vi "UE9 Config Comm.vi"() -> ()   [LabVIEW 2021]
panel:
  in  "Power Level":u8
  in  "Local ID":u8=1
  in  "DHCP Enabled":bool
  in  "Subnet":string="255.255.255.0"
  in  "Gateway":string="192.168.1.1"
  in  "PortB":u16=52361
  in  "PortA":u16=52360
  in  "IP Address":string="192.168.1.209"
  in  "FirstFound":bool=TRUE
  in  "ConnectionType":string="LJ_ctUSB"
  in  "Address":string="192.168.1.209"
  out "Error Message":string
  in  "error in":errorcluster
  out "error out":errorcluster
  # "Specify an IP address for Ethernet, or Local ID\nfor USB.  If FirstFound is selected, Local ID is\nignored for USB."
  # "Reset required for Ethernet parameters\nto take effect."
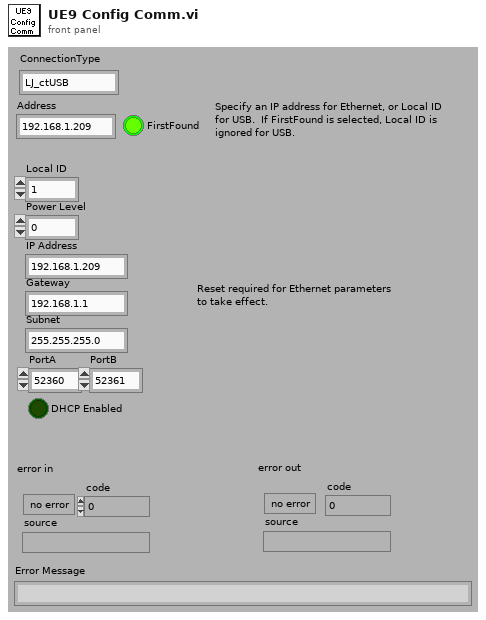
[diagram p1: front panel]
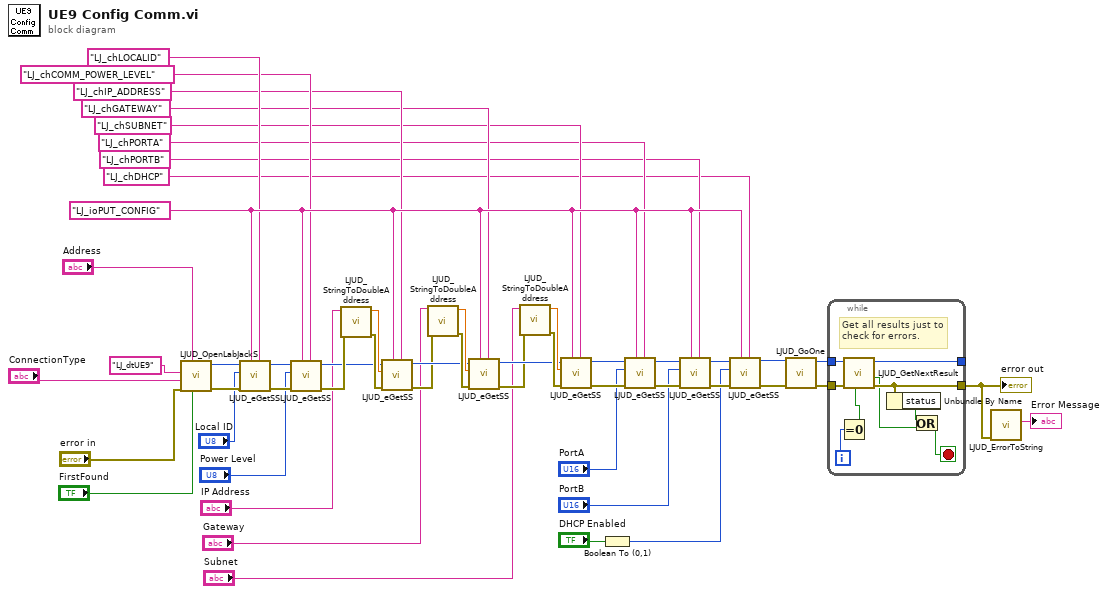
[diagram p0: block diagram]
diagram:
  w22 = "LJ_ioPUT_CONFIG" ("IOType")
  n1 = call "LJUD_OpenLabJackS.vi"("FirstFound"="FirstFound", "Address"="Address", "error in"="error in", "ConnectionType"="ConnectionType", "DeviceType"="LJ_dtUE9") -> ("error out"=w35:errorcluster, "Handle"=w38:i32)  [unwired: 4 in, 1 out]
  n2 = call "LJUD_eGetSS.vi"("Channel"="LJ_chLOCALID", "IOType"=w22, "error in"=w35, "Value Write"="Local ID", "Handle In"=w38) -> ("error out"=w34:errorcluster, "Handle Out"=w37:i32)  [unwired: 4 in, 1 out]
  n3 = call "LJUD_eGetSS.vi"("Channel"="LJ_chCOMM_POWER_LEVEL", "IOType"=w22, "error in"=w34, "Value Write"="Power Level", "Handle In"=w37) -> ("error out"=w28:errorcluster, "Handle Out"=w27:i32)  [unwired: 4 in, 1 out]
  n4 = call "LJUD_StringToDoubleAddress.vi"("error in"=w28, "String"="IP Address") -> ("error out"=w32:errorcluster, "Double Address"=w47:dbl)  [unwired: 8 in]
  n5 = call "LJUD_eGetSS.vi"("Channel"="LJ_chIP_ADDRESS", "IOType"=w22, "error in"=w32, "Value Write"=w47, "Handle In"=w27) -> ("error out"=w40:errorcluster, "Handle Out"=w42:i32)  [unwired: 4 in, 1 out]
  n6 = call "LJUD_StringToDoubleAddress.vi"("error in"=w40, "String"="Gateway") -> ("error out"=w45:errorcluster, "Double Address"=w46:dbl)  [unwired: 8 in]
  n7 = call "LJUD_eGetSS.vi"("Channel"="LJ_chGATEWAY", "IOType"=w22, "error in"=w45, "Value Write"=w46, "Handle In"=w42) -> ("error out"=w39:errorcluster, "Handle Out"=w41:i32)  [unwired: 4 in, 1 out]
  n8 = call "LJUD_StringToDoubleAddress.vi"("error in"=w39, "String"="Subnet") -> ("error out"=w44:errorcluster, "Double Address"=w43:dbl)  [unwired: 8 in]
  n9 = call "LJUD_eGetSS.vi"("Channel"="LJ_chSUBNET", "IOType"=w22, "error in"=w44, "Value Write"=w43, "Handle In"=w41) -> ("error out"=w31:errorcluster, "Handle Out"=w26:i32)  [unwired: 4 in, 1 out]
  n10 = Boolean To (0,1)(Boolean="DHCP Enabled") -> (0, 1=w7:i16)
  n11 = call "LJUD_eGetSS.vi"("Channel"="LJ_chPORTA", "IOType"=w22, "error in"=w31, "Value Write"="PortA", "Handle In"=w26) -> ("error out"=w23:errorcluster, "Handle Out"=w25:i32)  [unwired: 4 in, 1 out]
  n12 = call "LJUD_eGetSS.vi"("Channel"="LJ_chPORTB", "IOType"=w22, "error in"=w23, "Value Write"="PortB", "Handle In"=w25) -> ("error out"=w33:errorcluster, "Handle Out"=w36:i32)  [unwired: 4 in, 1 out]
  n13 = call "LJUD_eGetSS.vi"("Channel"="LJ_chDHCP", "IOType"=w22, "error in"=w33, "Value Write"=w7, "Handle In"=w36) -> ("error out"=w24:errorcluster, "Handle Out"=w6:i32)  [unwired: 4 in, 1 out]
  n14 = call "LJUD_GoOne.vi"("error in"=w24, "Handle In"=w6) -> ("error out"=w4:errorcluster, "Handle Out"=w3:i32)  [unwired: 8 in]
  n15 = while {
    tunnel: [w54] -> _
    tunnel: [w56] -> w5
    tunnel: w3 -> [w57]
    tunnel: w4 -> [w58]
    i -> [w53]
    stop <- w60 stop-if-true
    # "Get all results just to\ncheck for errors."
    n16 = Equal To 0?(x=w53) -> (x = 0?=w59:bool)
    n17 = call "LJUD_GetNextResult.vi"("GetFirst"=w59, "error in"=w58, "Handle In"=w57) -> ("error out"=w56:errorcluster, "LJE_NO_MORE_DATA_AVAILABLE"=w52:bool, "Handle Out"=w54:i32)  [unwired: 3 in, 3 out]
    n18 = Unbundle By Name(w56) -> ("status"=w55:bool)
    n19 = Or(x=w55, y=w52) -> (x .or. y?=w60:bool)
  }
  "error out" <- w5
  n20 = call "LJUD_ErrorToString.vi"("error in"=w5) -> ("String"=→"Error Message":string)  [unwired: 10 in]
